vi "Script Select UI.vi"(7 "Server Alias":string) -> ()   [LabVIEW 2013]
doc: "This VI allows the user to select a script to run on the Python side."
uses:
  LabVIEW Core/TS.lvlib
panel:
  in  "Clear Args":bool
  in  "Script Arguments (Optional)":string[](array[string])
  in  "Remote Python Script to Run":path=path "C:/Projects/IN110094 Python LabVIEW Interface/Python Core/Test Scripts"
  in  "Cancel Button":bool
  in  "OK Button":bool
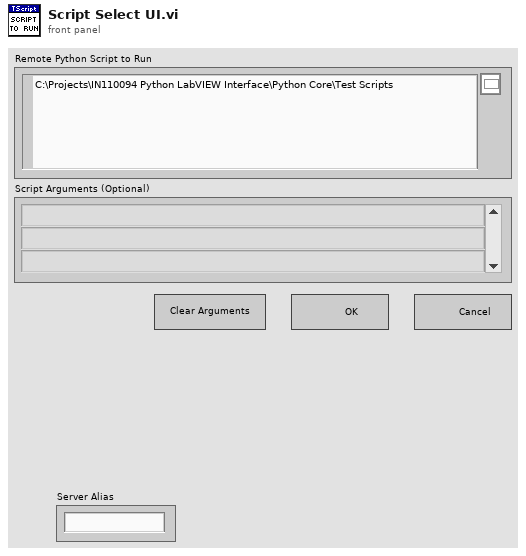
[diagram p1: front panel]
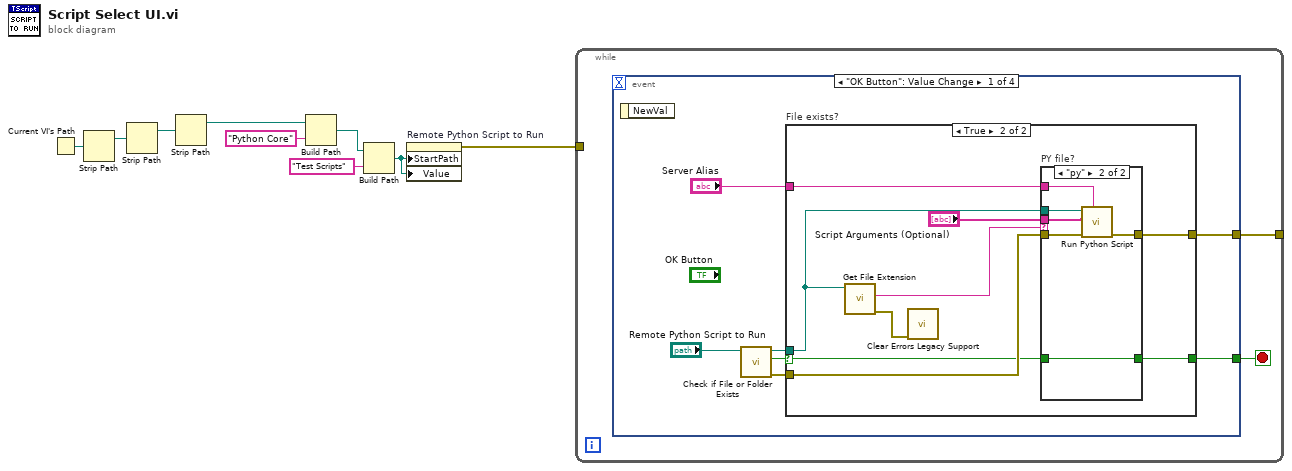
[diagram p0: block diagram]
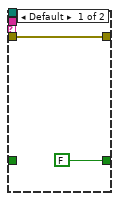
[diagram p3: hidden frame]
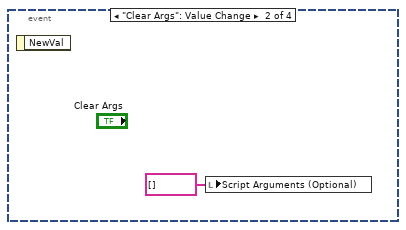
[diagram p4: hidden frame]
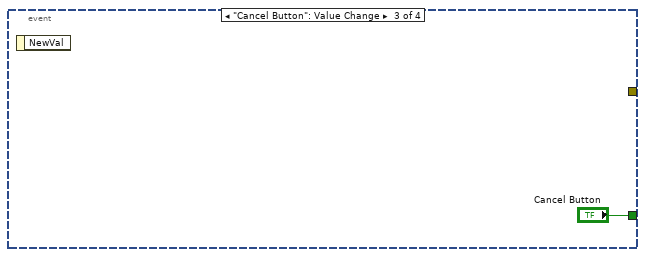
[diagram p5: hidden frame]
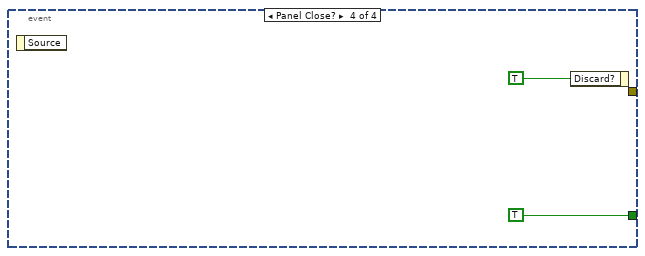
[diagram p6: hidden frame]
diagram:
  n1 = Current VI's Path() -> (path=w6:path)
  n2 = Strip Path(path=w6) -> (stripped path=w8:path)  [unwired: 1 out]
  n3 = Strip Path(path=w8) -> (stripped path=w9:path)  [unwired: 1 out]
  n4 = Strip Path(path=w9) -> (stripped path=w3:path)  [unwired: 1 out]
  n5 = Build Path(base path=w3, name or relative path="Python Core") -> (appended path=w4:path)
  n6 = Build Path(base path=w4, name or relative path="Test Scripts") -> (appended path=w1:path)
  n7 = property on="Remote Python Script to Run" class="Path"("StartPath"=w1, "Value"=w1) -> (error out=w2:errorcluster)  [unwired: 2 in, 1 out]
  n8 = while {
    tunnel: [w10] -> _
    tunnel: w2 -> [_]
    stop <- w11 stop-if-true
    n9 = event shown="[0] \"OK Button\": Value Change" {
      selector: _ -> [_ _ _ _]
      dyn-events: _ -> [_ _ _ _]
      timeout: _ -> [_ _ _ _]
      tunnel: [w15 _ "Cancel Button" TRUE ("Cancel Button")] -> w11
      tunnel: [w14 _ _ _] -> w10
      event "OK Button": Value Change {
        n10 = event-data() -> ()  [unwired: 1 in, 1 out]
        n11 = call <vilib>:"Check if File or Folder Exists.vi"("path"="Remote Python Script to Run") -> ("error out"=w13:errorcluster, "file or folder exists?"=w17:bool, "dup path"=w16:path)  [unwired: 8 in]
        n12 = case "File exists?" shown="True" w17 {
          selector: w17 -> [w19 w21]
          tunnel: w16 -> [_ w25]
          tunnel: [w19 w22] -> w15
          tunnel: [_ w27] -> w14
          tunnel: w13 -> [_ w26]
          tunnel: "Server Alias" -> [_ w20]
          frame False {
          }
          frame True {
            n13 = call <vilib>:"Get File Extension.vi"("file"=w25) -> ("error out"=w23:errorcluster, "lowercase file extension"=w24:string)  [unwired: 6 in, 3 out]
            n14 = call "Clear Errors Legacy Support.vi"("error in (no error)"=w23) -> ()  [unwired: 5 in, 2 out]
            n15 = case "PY file?" shown="\"py\"" w24 {
              tunnel: "Script Arguments (Optional)" -> [_ w36]
              tunnel: [w30 w35] -> w27
              tunnel: w26 -> [w30 w34]
              tunnel: w25 -> [_ w33]
              tunnel: [FALSE w32] -> w22
              tunnel: w21 -> [_ w32]
              tunnel: w20 -> [_ w31]
              frame Default {
              }
              frame "py" {
                n16 = call "Run Python Script.vi"("Server Alias"=w31, "error in (no error)"=w34, "Script Arguments (Optional)"=w36, "Absolute Python Script Path"=w33) -> ("error out"=w35:errorcluster)  [unwired: 7 in]
              }
            }
          }
        }
      }
      event "Clear Args": Value Change {
        n17 = event-data() -> ()  [unwired: 1 in, 1 out]
        n18 = local write "Script Arguments (Optional)"(string[] [] ("Script Arguments (Optional)")) -> ()
      }
      event "Cancel Button": Value Change {
        n19 = event-data() -> ()  [unwired: 1 in, 1 out]
      }
      event Panel Close? {
        n20 = event-data() -> ()  [unwired: 1 in, 1 out]
        n21 = event-data("Discard?"=TRUE) -> ()  [unwired: 1 in, 1 out]
      }
    }
  }
